vi "Batch Start Dialog Ex.vi"(1 "Curr GU":i32[](array[numeric]), 2 "Enabled Site":i32[](array[numeric])) -> (0 "OK?":bool)   [LabVIEW 2020, in "GUCalibration2.lvlib"]
uses:
  GUCalibration2.lvlib
  Controls/User Facing Msg Enum.ctl
panel:
  out "display":string
  in  "OK":bool
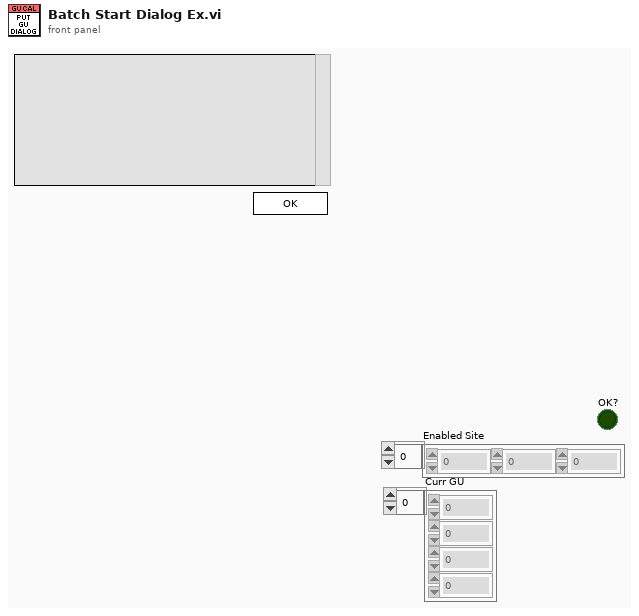
[diagram p1: front panel]
types:
  T1 = typedef "GUCalibration2.lvlib/User Facing Msg Enum.ctl" = enum16{"Invalid GU Number", "Select More GU", "Exceptional Lot End", "Not All Sites Test", "GU Arrange Error", "Put GU In Sites", "No Cal Site Offset Msg"}
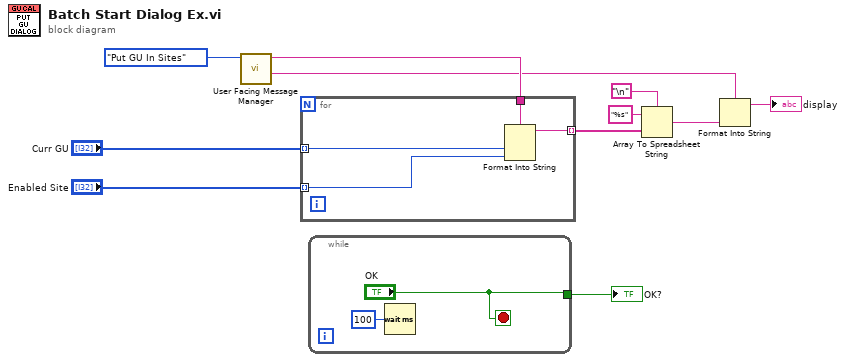
[diagram p0: block diagram]
diagram:
  n1 = call "User Facing Message Manager.vi"("User Facing Msg"=User_Facing_Msg_Enum."Put GU In Sites") -> ("Sub User Facing Msg Out"=w1:string, "User Facing Msg Out"=w2:string)  [unwired: 8 in, 1 out]
  n2 = for {
    tunnel: [w15] -> w8 mode=indexing
    tunnel: "Enabled Site" -> [w13] mode=indexing
    tunnel: "Curr GU" -> [w14] mode=indexing
    tunnel: w2 -> [w12]
    n3 = Format Into String(format string=w12, w14, w13) -> (resulting string=w15:string)  [unwired: 2 in, 1 out]
  }
  n4 = while {
    tunnel: ["OK"] -> w11
    stop <- "OK" stop-if-true
    n5 = Wait (ms)(milliseconds to wait=u32 100) -> ()  [unwired: 1 out]
  }
  "OK?" <- w11
  n6 = Array To Spreadsheet String(delimiter (Tab)="\n", array=w8, 3:"%s" ("format string")) -> (spreadsheet string=w5:string)
  n7 = Format Into String(format string=w1, w5) -> (resulting string=→"display":string)  [unwired: 2 in, 1 out]
